vi "Wire Nodes Together.vi"(7 "Shift Pressed?":bool, 8 "error in (no error)":errorcluster, 11 "VI Ref":refnum<vi>) -> (0 "error out":errorcluster, 3 "dup VI":refnum<vi>, 4 "Undo Fail?":bool)   [LabVIEW 2014]
doc: "Connects compatible terminals between multiple selected diagram objects. This shortcut will wire compatible data types between the objects in a left-to-right fashion. If [Shift] is also pressed, LabVIEW will perform a diagram cleanup of the selected objects after wiring them together.\n\nDefault Shortcut - [W]"
uses:
  <vilib>/Utility/traverseref.llb/TRef TravTarget.ctl
  <resource>/dialog/QuickDrop/plugins/_WireMultipleSupport/What to Wire.ctl
  <vilib>/Utility/traverseref.llb/VI Scripting - Traverse.lvlib
panel:
  in  "Undo Name":string="Wire Multiple Objects Together"
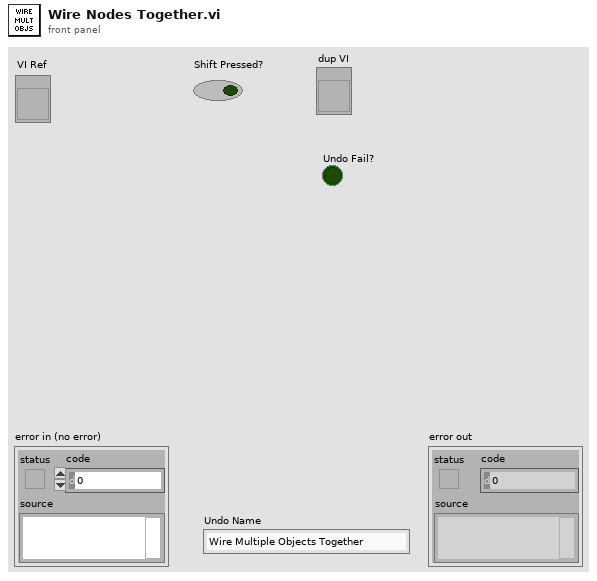
[diagram p1: front panel]
types:
  T1 = typedef "TRef TravTarget.ctl" = enum16{"FP", "BD", "Other"}
  T2 = typedef "What to Wire.ctl" = enum16{"node sinks", "node sources"}
  T3 = typedef "Node Terminal Info.ctl" = cluster{"Node Position (Left)":i32, "Node Ref":refnum<vi>, "Top Left":refnum<vi>, "Top Right":refnum<vi>, "Error Left":refnum<vi>, "Error Right":refnum<vi>}
  T4 = typedef "Available Non-Node.ctl" = cluster{"Left":i32, "Terminal":refnum<vi>}
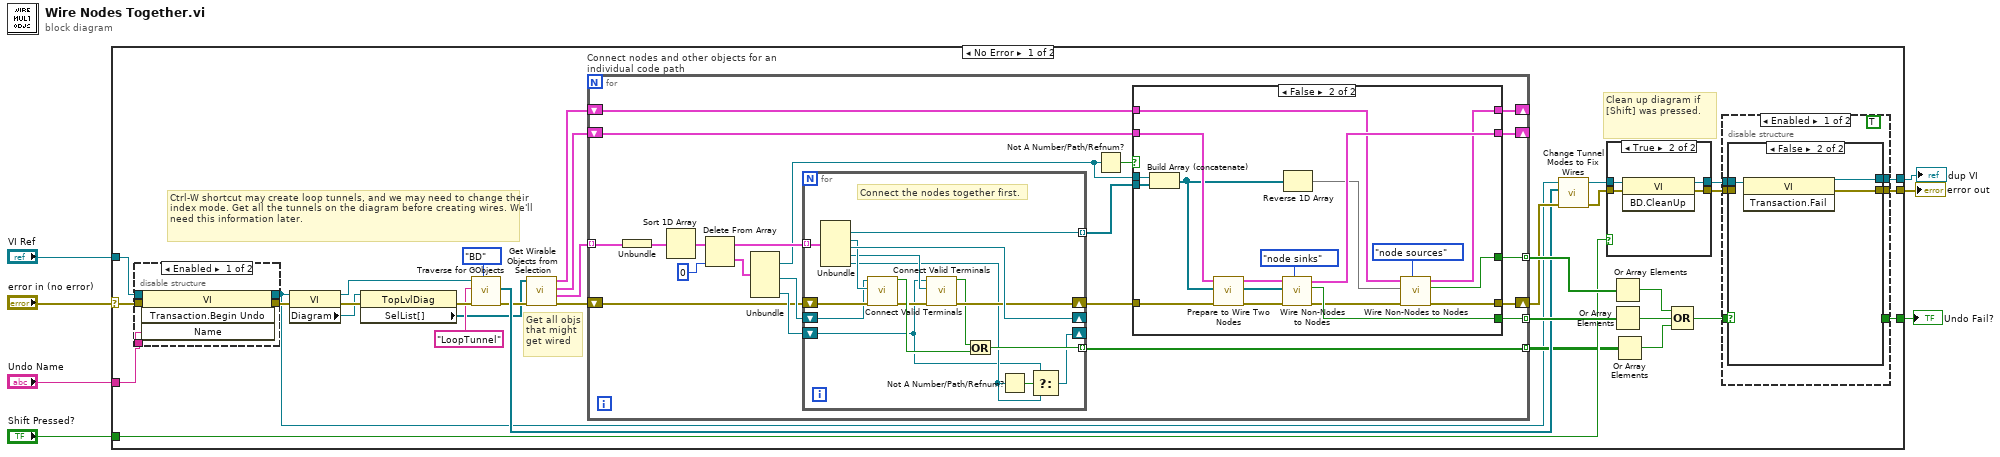
[diagram p0: block diagram]
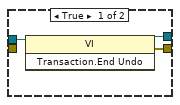
[diagram p2: hidden frame]
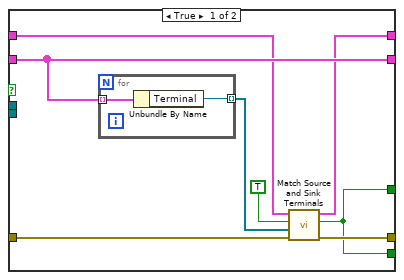
[diagram p5: hidden frame]
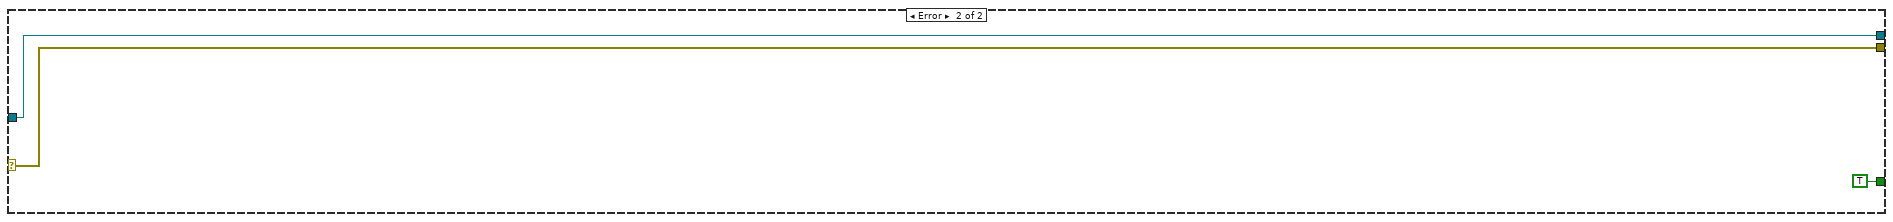
[diagram p7: hidden frame]
diagram:
  n1 = case shown="No Error" "error in (no error)" {
    selector: "error in (no error)" -> [w8 w136]
    tunnel: [w38 w136] -> w6
    tunnel: "VI Ref" -> [w41 w135]
    tunnel: "Shift Pressed?" -> [w29 _]
    tunnel: "Undo Name" -> [w40 _]
    tunnel: [w10 w135] -> w2
    tunnel: [w9 TRUE] -> w1
    frame No Error {
      # "Get all objs\nthat might\nget wired"
      # "Ctrl-W shortcut may create loop tunnels, and we may need to change their index mode. Get all the tunnels on the diagram before creating wires. We'll need this information later."
      # "Clean up diagram if [Shift] was pressed."
      n2 = disable-structure shown="Enabled" {
        disable-tunnel: w8 -> [w60 w62]
        disable-tunnel: w41 -> [w59 w61]
        disable-tunnel: w40 -> [w58 _]
        disable-tunnel: [w57 w62] -> w39
        disable-tunnel: [w56 w61] -> w13
        frame Enabled {
          n3 = invoke class="VI" method="Transaction.Begin Undo"(reference=w59, error in=w60, "Name"=w58) -> (reference out=w56:refnum<vi>, error out=w57:errorcluster)  [unwired: 1 in, 2 out]
        }
        frame Disabled {
        }
      }
      n4 = property class="VI"(reference=w13, error in=w39) -> (reference out=w23:refnum<vi>, error out=w37:errorcluster, "Diagram"=w36:refnum<vi>)
      n5 = property class="TopLvlDiag"(reference=w36, error in=w37) -> (error out=w35:errorcluster, "SelList[]"=w16:refnum<vi>[])  [unwired: 1 out]
      n6 = call <vilib>:"Traverse for GObjects.vi"("Traverse Target"=TRef_TravTarget."BD", "error in (no error)"=w35, "Class Name"="LoopTunnel", "VI Refnum"=w23) -> ("error out"=w20:errorcluster, "References"=w21:refnum<vi>[])  [unwired: 4 in, 2 out]
      n7 = call <resource>:"Get Wirable Objects from Selection.vi"("error in (no error)"=w20, "SelList[]"=w16) -> ("error out"=w15:errorcluster, "Parsed Selection List (Geographic Rows)"=w14:cluster{"Selection List":T3[]}[], "Controls, Constants, and Source Tunnels"=w17:T4[], "Indicators and Sink Tunnels"=w18:T4[])  [unwired: 6 in]
      n8 = for "Connect nodes and other objects for an individual code path" {
        tunnel: [w83] -> w33 mode=indexing
        tunnel: [w82] -> w30 mode=indexing
        tunnel: [w78] -> w19 mode=indexing
        shift-right: [w81] -> w27
        shift-left: w15 -> [w68]
        shift-right: [w67] -> _
        shift-left: w18 -> [w74]
        shift-right: [w66] -> _
        shift-left: w17 -> [w70]
        tunnel: w14 -> [w65] mode=indexing
        n9 = Unbundle(w65) -> ("Selection List"=w64:T3[])
        n10 = Sort 1D Array(array=w64) -> (sorted array=w77:T3[])
        n11 = Delete From Array(array=w77, index=0) -> (deleted portion=w80:T3, array with subset deleted=w79:T3[])  [unwired: 1 in]
        n12 = Unbundle(w80) -> ("Node Ref"=w71:refnum<vi>, "Top Right"=w73:refnum<vi>, "Error Right"=w72:refnum<vi>)  [unwired: 3 out]
        n13 = for {
          shift-right: [w119] -> w76
          shift-left: w68 -> [w123]
          tunnel: w79 -> [w127] mode=indexing
          shift-right: [w124] -> _
          shift-left: w73 -> [w116]
          tunnel: [w125] -> w78 mode=indexing
          tunnel: [w126] -> w75 mode=indexing
          shift-right: [w112] -> _
          shift-left: w72 -> [w113]
          # "Connect the nodes together first."
          n14 = Unbundle(w127) -> ("Node Ref"=w126:refnum<vi>, "Top Left"=w121:refnum<vi>, "Top Right"=w124:refnum<vi>, "Error Left"=w118:refnum<vi>, "Error Right"=w114:refnum<vi>)  [unwired: 1 out]
          n15 = call <resource>:"Connect Valid Terminals.vi"("error in (no error)"=w123, "Sink Term"=w121, "Source Term"=w116) -> ("error out"=w120:errorcluster, "Connection Made?"=w122:bool)  [unwired: 7 in]
          n16 = call <resource>:"Connect Valid Terminals.vi"("error in (no error)"=w120, "Sink Term"=w118, "Source Term"=w113) -> ("error out"=w119:errorcluster, "Connection Made?"=w117:bool)  [unwired: 7 in]
          n17 = Or(x=w117, y=w122) -> (x .or. y?=w125:bool)
          n18 = Not A Number/Path/Refnum?(number/path/refnum=w114) -> (NaN/Path/Refnum?=w115:bool)
          n19 = Select(t=w113, s=w115, f=w114) -> (s? t:f=w112:refnum<vi>)
        }
        n20 = Not A Number/Path/Refnum?(number/path/refnum=w71) -> (NaN/Path/Refnum?=w69:bool)
        n21 = case shown="False" w69 {
          tunnel: w76 -> [w90 w100]
          tunnel: w75 -> [_ w98]
          tunnel: [w84 w109] -> w83
          tunnel: [w84 w101] -> w82
          tunnel: w74 -> [w88 w103]
          tunnel: [w89 w106] -> w81
          tunnel: w71 -> [_ w111]
          tunnel: w70 -> [w91 w97]
          tunnel: [w87 w102] -> w67
          tunnel: [w91 w110] -> w66
          frame True {
            n22 = for {
              tunnel: w91 -> [w93] mode=indexing
              tunnel: [w92] -> w86 mode=indexing
              n23 = Unbundle By Name(w93) -> ("Terminal"=w92:refnum<vi>)
            }
            n24 = call <resource>:"Match Source and Sink Terminals.vi"("error in (no error)"=w90, "Node Terminals"=w86, "Node Sources?"=TRUE, "Available Non-Nodes in"=w88) -> ("error out"=w89:errorcluster, "Any Changes?"=w84:bool, "Available Non-Nodes out"=w87:T4[])  [unwired: 5 in]
          }
          frame False {
            n25 = Build Array (concatenate)(w111, w98) -> (w95:refnum<vi>[])
            n26 = call <resource>:"Prepare to Wire Two Nodes.vi"("error in (no error)"=w100, "Nodes"=w95, "Available Non-Nodes in"=w97) -> ("error out"=w99:errorcluster, "dup Nodes"=w94:refnum<vi>[], "Available Non-Nodes out"=w96:T4[])  [unwired: 6 in]
            n27 = call <resource>:"Wire Non-Nodes to Nodes.vi"("What to Wire"=What_to_Wire."node sinks", "error in (no error)"=w99, "Nodes"=w94, "Available Non-Nodes in"=w96) -> ("error out"=w107:errorcluster, "Any Changes?"=w109:bool, "Available Non-Nodes out"=w110:T4[])  [unwired: 5 in]
            n28 = Reverse 1D Array(array=w95) -> (reversed array=w104:refnum<vi>[])
            n29 = call <resource>:"Wire Non-Nodes to Nodes.vi"("What to Wire"=What_to_Wire."node sources", "error in (no error)"=w107, "Nodes"=w104, "Available Non-Nodes in"=w103) -> ("error out"=w106:errorcluster, "Any Changes?"=w101:bool, "Available Non-Nodes out"=w102:T4[])  [unwired: 5 in]
          }
        }
      }
      n30 = call <resource>:"Change Tunnel Modes to Fix Wires.vi"("error in (no error)"=w27, "All Tunnels (before wiring)"=w21, "VI"=w13) -> ("error out"=w26:errorcluster, "dup VI"=w12:refnum<vi>)  [unwired: 7 in]
      n31 = case shown="True" w29 {
        tunnel: w26 -> [w129 w133]
        tunnel: [w129 w132] -> w11
        tunnel: w12 -> [w128 w131]
        tunnel: [w128 w130] -> w28
        frame False {
        }
        frame True {
          n32 = invoke class="VI" method="BD.CleanUp"(reference=w131, error in=w133) -> (reference out=w130:refnum<vi>, error out=w132:errorcluster)  [unwired: 1 in, 1 out]
        }
      }
      n33 = Or Array Elements(Boolean array=w30) -> (logical OR=w31:bool)
      n34 = Or Array Elements(Boolean array=w33) -> (logical OR=w32:bool)
      n35 = Or Array Elements(Boolean array=w19) -> (logical OR=w22:bool)
      n36 = Compound Arithmetic op=OR(w31, w32, w22) -> (w34:bool)
      n37 = disable-structure shown="Enabled" {
        disable-tunnel: [w46 w55] -> w38
        disable-tunnel: w34 -> [w45 w53]
        disable-tunnel: w28 -> [w44 w54]
        disable-tunnel: w11 -> [w43 w55]
        disable-tunnel: [w42 w54] -> w10
        disable-tunnel: [_ w53] -> w9
        frame Enabled {
          (unwired) TRUE
          n38 = case shown="False" w45 {
            tunnel: w44 -> [w48 w51]
            tunnel: [w49 w52] -> w46
            tunnel: w43 -> [_ _]
            tunnel: [w47 w50] -> w42
            frame True {
              n39 = invoke class="VI" method="Transaction.End Undo"(reference=w48) -> (reference out=w47:refnum<vi>, error out=w49:errorcluster)  [unwired: 2 in, 1 out]
            }
            frame False {
              n40 = invoke class="VI" method="Transaction.Fail"(reference=w51) -> (reference out=w50:refnum<vi>, error out=w52:errorcluster)  [unwired: 2 in, 1 out]
            }
          }
        }
        frame Disabled {
        }
      }
    }
    frame Error {
    }
  }
  "error out" <- w6
  "dup VI" <- w2
  "Undo Fail?" <- w1
